vi "durationScalar.vi"(4 "Duration":cluster{"secs":i32, "nsecs":i32}, 5 "msg in":string) -> (2 "msg out":string)   [LabVIEW 2014]
doc: "Flattens a duration scaler into a message"
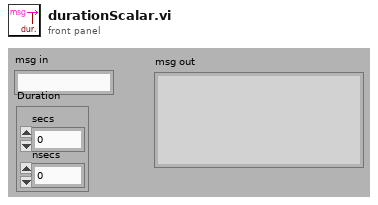
[diagram p1: front panel]
types:
  T1 = enum16{"big-endian, network order", "native, host order", "little-endian"}
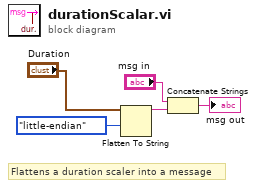
[diagram p0: block diagram]
diagram:
  # "Flattens a duration scaler into a message"
  n1 = Flatten To String(anything="Duration", byte order (0:big-endian, network order)=T1."little-endian") -> (data string=w4:string)  [unwired: 2 in, 2 out]
  n2 = Concatenate Strings("msg in", w4) -> (→"msg out":string)
